vi "Quinn's First Interpolation method.vi"(7 "FFT  spectrum":dbl[](array[numeric]), 8 "FFT array Im":dbl[](array[numeric]), 11 "FFT array Re":dbl[](array[numeric])) -> (0 "max index(es)":i32, 3 "Index Bin":dbl)   [LabVIEW 2014]
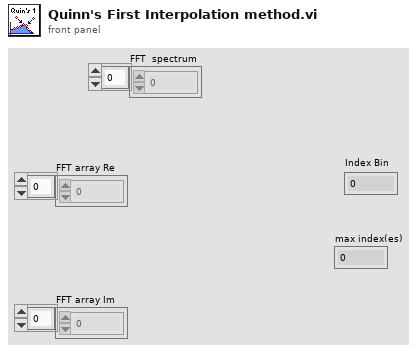
[diagram p1: front panel]
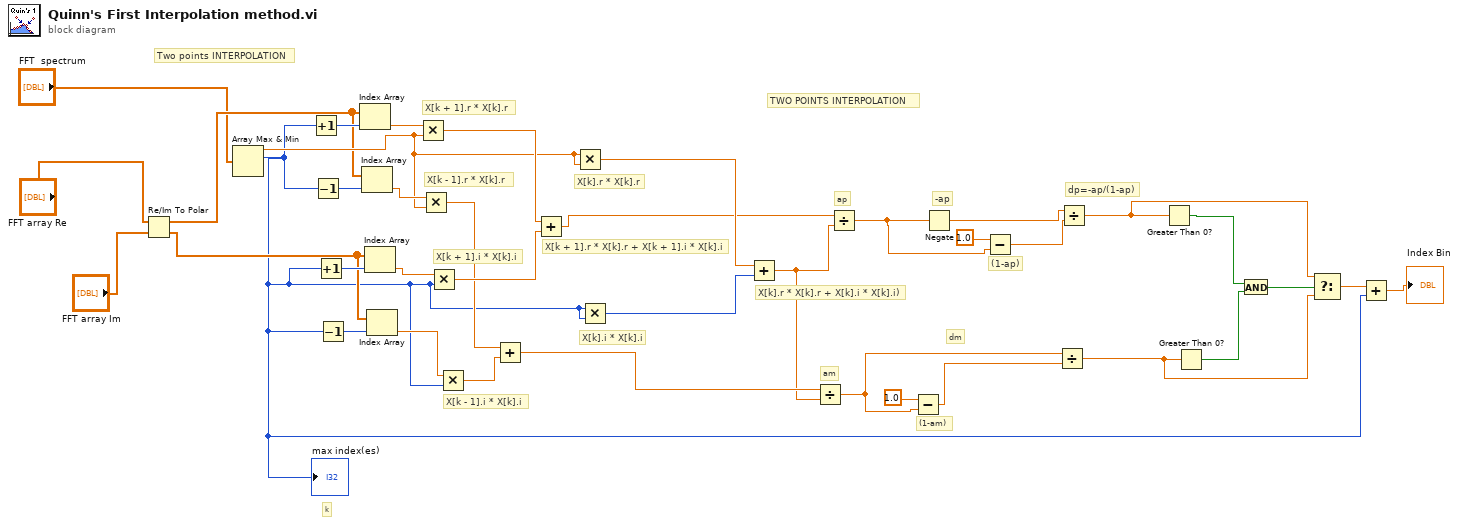
[diagram p0: block diagram]
diagram:
  # "TWO POINTS INTERPOLATION"
  # "Two points INTERPOLATION"
  # "k"
  # "dm"
  # "(1-am)"
  # "am"
  # "X[k - 1].r * X[k].r"
  # "X[k - 1].i * X[k].i"
  # "dp=-ap/(1-ap)"
  # "(1-ap)"
  # "-ap"
  # "ap"
  # "X[k].r * X[k].r + X[k].i * X[k].i)"
  # "X[k + 1].r * X[k].r + X[k + 1].i * X[k].i"
  # "X[k].r * X[k].r"
  # "X[k].i * X[k].i"
  # "X[k + 1].i * X[k].i"
  # "X[k + 1].r * X[k].r"
  n1 = Re/Im To Polar(2:"FFT array Im", 3:"FFT array Re") -> (0:w4:dbl[], 1:w5:dbl[])
  n2 = Array Max & Min(array="FFT  spectrum") -> (max value=w21:dbl, max index (indices)=w3:i32)  [unwired: 2 out]
  "max index(es)" <- w3
  n3 = Increment(x=w3) -> (x+1=w38:i32)
  n4 = Decrement(x=w3) -> (x-1=w37:i32)
  n5 = Increment(x=w3) -> (x+1=w35:i32)
  n6 = Decrement(x=w3) -> (x-1=w36:i32)
  n7 = Index Array(array=w5, index=w38) -> (element=w34:dbl)
  n8 = Index Array(array=w5, index=w37) -> (element=w22:dbl)
  n9 = Index Array(array=w4, index=w35) -> (element=w33:dbl)
  n10 = Index Array(array=w4, index=w36) -> (element=w23:dbl)
  n11 = Multiply(x=w34, y=w21) -> (x*y=w32:dbl)
  n12 = Multiply(x=w22, y=w21) -> (x*y=w19:dbl)
  n13 = Multiply(x=w33, y=w3) -> (x*y=w31:dbl)
  n14 = Multiply(x=w23, y=w3) -> (x*y=w20:dbl)
  n15 = Add(x=w19, y=w20) -> (x+y=w18:dbl)
  n16 = Add(x=w32, y=w31) -> (x+y=w28:dbl)
  n17 = Multiply(x=w21, y=w21) -> (x*y=w29:dbl)
  n18 = Multiply(x=w3, y=w3) -> (x*y=w30:i32)
  n19 = Add(x=w29, y=w30) -> (x+y=w17:dbl)
  n20 = Divide(x=w18, y=w17) -> (x/y=w15:dbl)
  n21 = Divide(x=w28, y=w17) -> (x/y=w26:dbl)
  n22 = Subtract(x=1.0, y=w15) -> (x-y=w14:dbl)
  n23 = Negate(x=w26) -> (-x=w25:dbl)
  n24 = Subtract(x=1.0, y=w26) -> (x-y=w24:dbl)
  n25 = Divide(x=w15, y=w14) -> (x/y=w9:dbl)
  n26 = Divide(x=w25, y=w24) -> (x/y=w10:dbl)
  n27 = Greater Than 0?(x=w10) -> (x > 0?=w12:bool)
  n28 = Greater Than 0?(x=w9) -> (x > 0?=w13:bool)
  n29 = And(x=w12, y=w13) -> (x .and. y?=w11:bool)
  n30 = Select(t=w10, s=w11, f=w9) -> (s? t:f=w8:dbl)
  n31 = Add(x=w8, y=w3) -> (x+y=→"Index Bin":dbl)
